vi "PicohrdlOpenUnit.vi"(8 "error in (no error)":errorcluster) -> (0 "error out":errorcluster, 3 "Handle out":i16, 4 "minAdc":i32, 6 "maxAdc":i32)   [LabVIEW 2010]
doc: "Calls HRDLOpenUnit()"
uses:
  PicoHRDL.dll
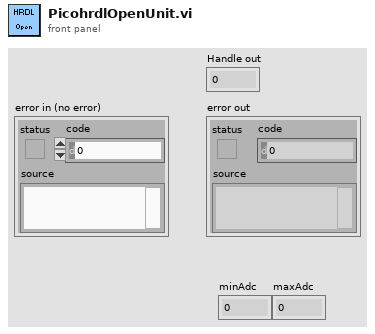
[diagram p1: front panel]
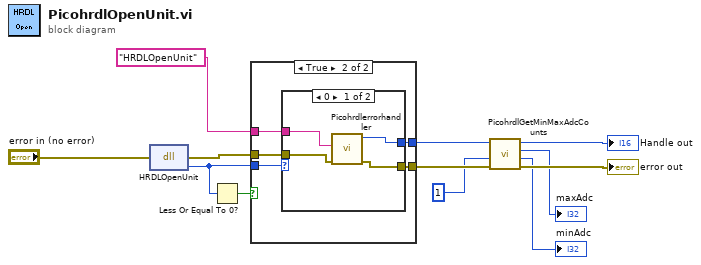
[diagram p0: block diagram]
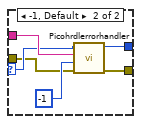
[diagram p3: hidden frame]
diagram:
  n1 = dll-call lib="PicoHRDL.dll" fn="HRDLOpenUnit"(error in="error in (no error)") -> (error out=w8:errorcluster, "handle"=w11:i16)  [unwired: 2 in, 1 out]
  n2 = Less Or Equal To 0?(x=w11) -> (x <= 0?=w10:bool)
  n3 = case shown="True" w10 {
    tunnel: [w14 w19] -> w6
    tunnel: "HRDLOpenUnit" ("API function") -> [_ w18]
    tunnel: w11 -> [w14 w17]
    tunnel: [w13 w16] -> w7
    tunnel: w8 -> [w13 w15]
    frame False {
    }
    frame True {
      n4 = case shown="0" w17 {
        selector: w17 -> [_ w26]
        tunnel: [w23 w29] -> w19
        tunnel: w18 -> [w22 w28]
        tunnel: [w21 w25] -> w16
        tunnel: w15 -> [w20 w24]
        frame 0 {
          n5 = call "Picohrdlerrorhandler.vi"("API function"=w22, "error in (no error)"=w20) -> ("Handle out"=w23:i16, "error out"=w21:errorcluster)  [unwired: 7 in]
        }
        frame -1, Default {
          n6 = call "Picohrdlerrorhandler.vi"("Handle in"=w26, "API function"=w28, "Return"=i16 -1, "error in (no error)"=w24) -> ("Handle out"=w29:i16, "error out"=w25:errorcluster)  [unwired: 5 in]
        }
      }
    }
  }
  n7 = call "PicohrdlGetMinMaxAdcCounts.vi"("error in (no error)"=w7, "channel"=i16 1, "handle in"=w6) -> ("error out"=→"error out":errorcluster, "minAdc"=→"minAdc":i32, "maxAdc"=→"maxAdc":i32, "handle out"=→"Handle out":i16)  [unwired: 5 in]
